vi "Autonomous Independent.vi"() -> ()   [LabVIEW 2018]
doc: "This VI is called when autonomous begins, and will automatically be terminated when autonomous ends. You can carry out timed or sensor driven robot movement independently without needing to return to the caller."
uses:
  <vilib>/Rock Robotics/WPI/Solenoid/WPI_SolenoidValue.ctl
  <vilib>/Rock Robotics/WPI/Utilities/WPI_GetSetVariantRefNum.vi
  <vilib>/Rock Robotics/Network Tables/NT Read String.vi
  <vilib>/Rock Robotics/WPI/RobotDrive/WPI_RobotDriveArcadeDrive_Standard(NoSaturation).vi
  <vilib>/Rock Robotics/Network Tables/NT Write Numeric Array.vi
  <vilib>/Rock Robotics/WPI/Solenoid/WPI_SolenoidSetEnum.vi
panel:
  in  "STOP?":bool
  out "Current Movement, for debugging":T1 {"Y Joystick Value" scale=1.0..-1.0; "X Joystick Value" scale=-1.0..1.0}
  in  "Array of robot movements":T2(array[cluster])=[{"X Joystick Value"=-0.010101010101010055, "Y Joystick Value"=0.0, "Delay (sec)"=0.1, "Movement Name"="turn"}, {"X Joystick Value"=-0.010101010101010055, "Y Joystick Value"=-0.40816326530612224, "Delay (sec)"=2.0, "Movement Name"="Drive Up"}, {"X Joystick Value"=0.0, "Y Joystick Value"=0.0, "Delay (sec)"=0.0, "Movement Name"="STOP"}] {"Y Joystick Value" scale=1.0..-1.0; "X Joystick Value" scale=-1.0..1.0}
  # "Be sure to right-click and choose Data Operations>>Make Current Value default if you want to save the array values with the VI"
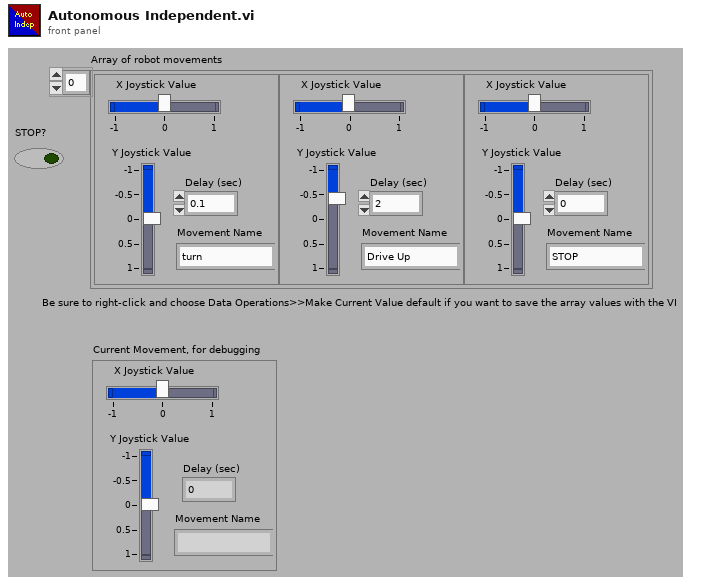
[diagram p1: front panel]
types:
  T1 = cluster{"X Joystick Value":dbl, "Y Joystick Value":dbl, "Delay (sec)":dbl, "Movement Name":string}
  T2 = cluster{"X Joystick Value":dbl, "Y Joystick Value":dbl, "Delay (sec)":dbl, "Movement Name":string}[]
  T3 = typedef "WPI_JoystickDevRef.ctl" = cluster{"Device":T4}
  T4 = typedef "WPI_JoystickDeviceEnum.ctl" = enum16{"USB 0", "USB 1", "USB 2", "USB 3", "USB 4", "USB 5"}
  T5 = typedef "WPI_SolenoidDevRef.ctl" = cluster{"DevStatus":errorcluster, "Pneumatics Control Module":u8, "Forward Solenoid Channel":T6, "Reverse Solenoid Channel":T6}
  T6 = typedef "WPI_SolenoidChannel.ctl" = enum8{"Solenoid 0", "Solenoid 1", "Solenoid 2", "Solenoid 3", "Solenoid 4", "Solenoid 5", "Solenoid 6", "Solenoid 7", "Invalid"}
  T7 = typedef "WPI_RobotDriveDevRef.ctl" = cluster{"DevStatus":errorcluster, "Motors[]":T8[], "Square Inputs":bool, "Max Output":dbl}
  T8 = typedef "WPI_MotorControlDeviceRef.ctl" = cluster{"DeviceStatus":errorcluster, "Type":T9, "PWM":cluster{"PWM Channel":T10, "DeadBand":T11}, "CAN":cluster{"Device Number":u8, "SetOutput VI Ref":variant, "GetOutput VI Ref":variant, "Enable VI Ref":variant, "Disable VI Ref":variant, "Data":variant}, "Invert":bool, "DIO PWM":cluster{"PWM \"Enable\" Channel":T10, "DIOChannel":T12, "PWM Rate":dbl}}
  T9 = typedef "WPI_MotorControlType.ctl" = enum16{"PWM", "CAN", "DIO PWM"}
  T10 = typedef "FPGA_DIOPWMChannel.ctl" = enum8{"PWM 0", "PWM 1", "PWM 2", "PWM 3", "PWM 4", "PWM 5", "PWM 6", "PWM 7", "PWM 8", "PWM 9", "PWM MXP 0", "PWM MXP 1", "PWM MXP 2", "PWM MXP 3", "PWM MXP 4", "PWM MXP 5", "PWM MXP 6", "PWM MXP 7", "PWM MXP 8", "PWM MXP 9", "Invalid"}
  T11 = typedef "WPI_PWMDeadband.ctl" = cluster{"Name":string, "maxPositivePwm":i32, "minPositivePwm":i32, "centerPwm":i32, "maxNegativePwm":i32, "minNegativePwm":i32, "angularRange":u16}
  T12 = typedef "FPGA_DIOChannel.ctl" = enum8{"DIO 0", "DIO 1", "DIO 2", "DIO 3", "DIO 4", "DIO 5", "DIO 6", "DIO 7", "DIO 8", "DIO 9", "DIO MXP 0", "DIO MXP 1", "DIO MXP 2", "DIO MXP 3", "DIO MXP 4", "DIO MXP 5", "DIO MXP 6", "DIO MXP 7", "DIO MXP 8", "DIO MXP 9", "DIO MXP 10", "DIO MXP 11", "DIO MXP 12", "DIO MXP 13", "DIO MXP 14", "DIO MXP 15", "SPI Port CS1", "SPI Port CS2", "SPI Port CS3", "SPI Port MISO", "SPI Port MOSI", "Invalid"}
  T13 = typedef "WPI_ServoDeviceRef.ctl" = cluster{"DeviceStatus":errorcluster, "PWM Channel":T10, "DeadBand":T11}
  T14 = typedef "WPI_SolenoidValue.ctl" = enum16{"Off", "On", "Forward", "Reverse"}
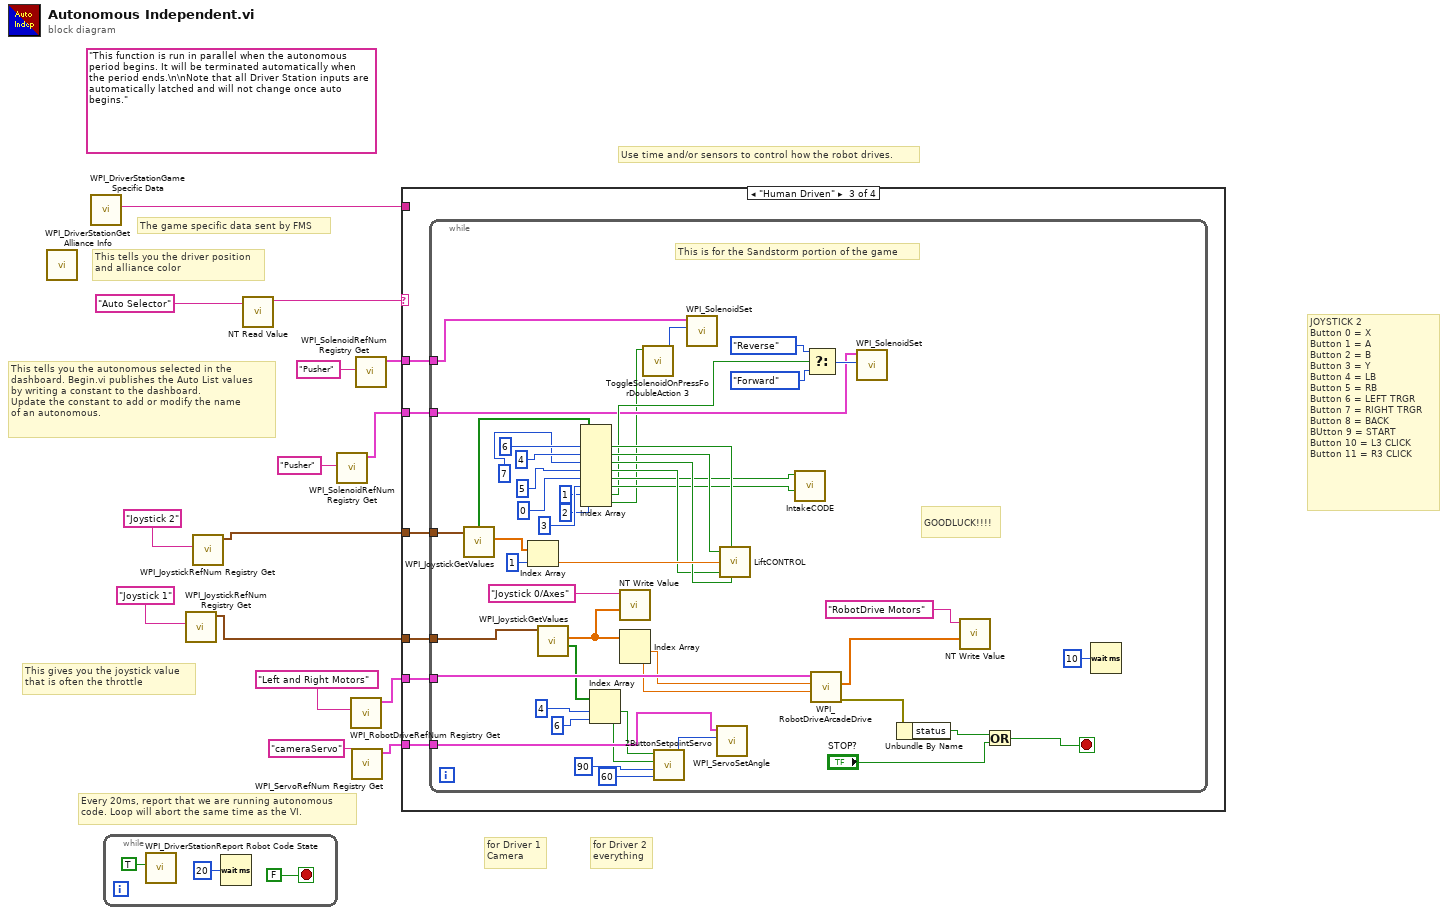
[diagram p0: block diagram]
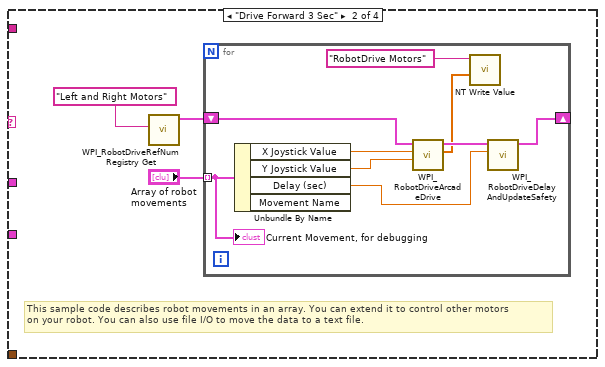
[diagram p3: hidden frame]
diagram:
  (unwired) "This function is run in parallel when the autonomous period begins. It will be terminated automatically when the period ends.\n\nNote that all Driver Station inputs are automatically latched and will not change once auto begins."
  # "JOYSTICK 2\nButton 0 = X\nButton 1 = A\nButton 2 = B\nButton 3 = Y\nButton 4 = LB \nButton 5 = RB\nButton 6 = LEFT TRGR \nButton 7 = RIGHT TRGR \nButton 8 = BACK\nBUtton 9 = START\nButton 10 = L3 CLICK\nButton 11 = R3 CLICK"
  # "for Driver 2\neverything"
  # "for Driver 1\nCamera"
  # "The game specific data sent by FMS"
  # "This tells you the autonomous selected in the \ndashboard. Begin.vi publishes the Auto List values\nby writing a constant to the dashboard.\nUpdate the constant to add or modify the name\nof an autonomous."
  # "Every 20ms, report that we are running autonomous\ncode. Loop will abort the same time as the VI."
  # "This gives you the joystick value\nthat is often the throttle"
  # "Use time and/or sensors to control how the robot drives."
  # "This tells you the driver position\nand alliance color"
  n1 = call <vilib>:"WPI_DriverStationGet Alliance Info.vi"() -> ()  [unwired: 12 out]
  n2 = call <vilib>:"WPI_DriverStationGame Specific Data.vi"() -> ("Game Specific Data"=w12:string)  [unwired: 11 in]
  n3 = while {
    stop <- FALSE stop-if-true
    n4 = call <vilib>:"WPI_DriverStationReport Robot Code State.vi"("Autonomous"=TRUE) -> ()  [unwired: 10 in, 1 out]
    n5 = Wait (ms)(milliseconds to wait=u32 20) -> ()  [unwired: 1 out]
  }
  n6 = call <vilib>:"WPI_JoystickRefNum Registry Get.vi"("refnum name"="Joystick 1") -> ("JoystickDevRef"=w9:T3)  [unwired: 1 in, 9 out]
  n7 = call <vilib>:"WPI_JoystickRefNum Registry Get.vi"("refnum name"="Joystick 2") -> ("JoystickDevRef"=w7:T3)  [unwired: 1 in, 9 out]
  n8 = call-poly <vilib>:"NT Read Value.vi"("Name"="Auto Selector") -> ("String"=w13:string)  [unwired: 9 in, 1 out]
  n9 = call <vilib>:"WPI_SolenoidRefNum Registry Get.vi"("refnum name"="Pusher") -> ("SolenoidDevRef"=w4:T5)  [unwired: 9 in, 1 out]
  n10 = call <vilib>:"WPI_RobotDriveRefNum Registry Get.vi"("refnum name"="Left and Right Motors") -> ("RobotDriveDevRef"=w10:T7)  [unwired: 1 in, 9 out]
  n11 = call <vilib>:"WPI_ServoRefNum Registry Get.vi"("refnum name"="cameraServo") -> ("ServoDeviceRef"=w5:T13)  [unwired: 9 in, 1 out]
  n12 = call <vilib>:"WPI_SolenoidRefNum Registry Get.vi"("refnum name"="Pusher") -> ("SolenoidDevRef"=w1:T5)  [unwired: 9 in, 1 out]
  n13 = case shown="\"Human Driven\"" w13 {
    tunnel: w12 -> [_ _ _ _]
    tunnel: w10 -> [_ _ w36 _]
    tunnel: w9 -> [_ _ w35 _]
    tunnel: w7 -> [_ _ w34 _]
    tunnel: w5 -> [_ _ w33 _]
    tunnel: w4 -> [_ _ w32 _]
    tunnel: w1 -> [_ _ w31 _]
    frame Default {
      # "You can put your main auto here, or you can right-click on the case and make any\nother frame be the default case."
      # "This is the frame that will execute if no selection is made, or if it is not recognized"
    }
    frame "Drive Forward 3 Sec" {
      # "This sample code describes robot movements in an array. You can extend it to control other motors\non your robot. You can also use file I/O to move the data to a text file."
      n14 = call <vilib>:"WPI_RobotDriveRefNum Registry Get.vi"("refnum name"="Left and Right Motors") -> ("RobotDriveDevRef"=w20:T7)  [unwired: 1 in, 9 out]
      n15 = for {
        shift-right: [w28] -> _
        shift-left: w20 -> [w29]
        tunnel: "Array of robot movements" -> [w24] mode=indexing
        n16 = Unbundle By Name(w24) -> ("X Joystick Value"=w27:dbl, "Y Joystick Value"=w26:dbl, "Delay (sec)"=w25:dbl)  [unwired: 1 out]
        n17 = call-poly <vilib>:"WPI_RobotDriveArcadeDrive.vi"("Y axis value"=w26, "X axis value"=w27, "RobotDriveDevRef"=w29) -> ("Motor Values"=w22:dbl[], "RobotDriveDevRef"=w30:T7)  [unwired: 1 in, 6 out]
        n18 = call-poly <vilib>:"NT Write Value.vi"("Numeric Array"=w22, "Name"="RobotDrive Motors") -> ()  [unwired: 9 in, 1 out]
        n19 = call <vilib>:"WPI_RobotDriveDelayAndUpdateSafety.vi"("Delay (s)"=w25, "RobotDriveDevRef"=w30) -> ("RobotDriveDevRef 2"=w28:T7)  [unwired: 8 in, 1 out]
        "Current Movement, for debugging" <- w24
      }
    }
    frame "Human Driven" {
      n20 = while {
        tunnel: w36 -> [w83]
        tunnel: w35 -> [w80]
        tunnel: w34 -> [w77]
        tunnel: w33 -> [w63]
        tunnel: w32 -> [w42]
        tunnel: w31 -> [w39]
        stop <- w53 stop-if-true
        # "GOODLUCK!!!!"
        # "This is for the Sandstorm portion of the game"
        n21 = call <vilib>:"WPI_JoystickGetValues.vi"("JoystickDevRef"=w77) -> ("Buttons"=w76:bool[], "Axes"=w75:dbl[])  [unwired: 6 in, 3 out]
        n22 = Index Array(array=w75, index=1) -> (element=w73:dbl)
        n23 = call <vilib>:"WPI_JoystickGetValues.vi"("JoystickDevRef"=w80) -> ("Buttons"=w60:bool[], "Axes"=w82:dbl[])  [unwired: 6 in, 3 out]
        n24 = Index Array(array=w76, index #1=6 ("index"), index #2=4 ("index"), index #3=7 ("index"), index #4=5 ("index"), index #5=0 ("index"), index #6=3 ("index"), index #7=1 ("index"), index #8=2 ("index")) -> (element #1=w70:bool, element #2=w69:bool, element #3=w67:bool, element #4=w65:bool, element #5=w49:bool, element #6=w48:bool, element #7=w43:bool, element #8=w37:bool)
        n25 = Index Array(array=w60, index #1=4 ("index"), index #2=6 ("index")) -> (element #1=w57:bool, element #2=w56:bool)
        n26 = call-poly <vilib>:"NT Write Value.vi"("Numeric Array"=w82, "Name"="Joystick 0/Axes") -> ()  [unwired: 9 in, 1 out]
        n27 = Index Array(array=w82) -> (element #1=w79:dbl, element #2=w78:dbl)  [unwired: 2 in]
        n28 = call "ToggleSolenoidOnPressForDoubleAction 3.vi"("Button"=w37) -> ("Value"=w40:T14)  [unwired: 10 in]
        n29 = call "2ButtonSetpointServo.vi"("Setpoint B"=60 ("Setpoint A"), "Setpoint A"=90, "Button 1"=w56, "Button 2"=w57) -> ("Value Out"=w64:i32)  [unwired: 7 in]
        n30 = call-poly <vilib>:"WPI_SolenoidSet.vi"("Value"=w40, "SolenoidDevRef"=w39) -> ()  [unwired: 8 in, 2 out]
        n31 = call <vilib>:"WPI_ServoSetAngle.vi"("Angle"=w64, "ServoDeviceRef"=w63) -> ()  [unwired: 8 in, 2 out]
        n32 = call "LiftCONTROL.vi"("Left Bumper"=w69, "Left Trigger"=w70, "Manual Control"=w73, "Right Bumper"=w65, "Right Trigger"=w67) -> ()  [unwired: 2 in]
        n33 = call "IntakeCODE.vi"("Intake Button B"=w48, "Intake Button A"=w49) -> ()  [unwired: 9 in, 1 out]
        n34 = Select(t=WPI_SolenoidValue."Reverse" ("Value"), s=w43, f=WPI_SolenoidValue."Forward" ("Value")) -> (s? t:f=w45:T14)
        n35 = call-poly <vilib>:"WPI_RobotDriveArcadeDrive.vi"("Y axis value"=w78, "X axis value"=w79, "RobotDriveDevRef"=w83) -> ("error out"=w55:errorcluster, "Motor Values"=w84:dbl[])  [unwired: 1 in, 6 out]
        n36 = call-poly <vilib>:"WPI_SolenoidSet.vi"("Value"=w45, "SolenoidDevRef"=w42) -> ()  [unwired: 8 in, 2 out]
        n37 = Unbundle By Name(w55) -> ("status"=w54:bool)
        n38 = call-poly <vilib>:"NT Write Value.vi"("Numeric Array"=w84, "Name"="RobotDrive Motors") -> ()  [unwired: 9 in, 1 out]
        n39 = Or(x=w54, y="STOP?") -> (x .or. y?=w53:bool)
        n40 = Wait (ms)(milliseconds to wait=u32 10) -> ()  [unwired: 1 out]
      }
    }
    frame "Your Turn" {
    }
  }
